vi "Init.vi"(8 "error in (no error)":errorcluster, 10 "Variant":variant, 11 "SpinCoater in":refnum<class "SpinCoater.lvclass">) -> (0 "error out":errorcluster, 3 "SpinCoater out":refnum<class "SpinCoater.lvclass">)   [LabVIEW 2020, in "SpinCoater.lvclass"]
uses:
  <instrlib>/Classes/SpinCoater/SpinCoater.lvclass
  <vilib>/Instr/_visa.llb/VISA Configure Serial Port (Instr).vi
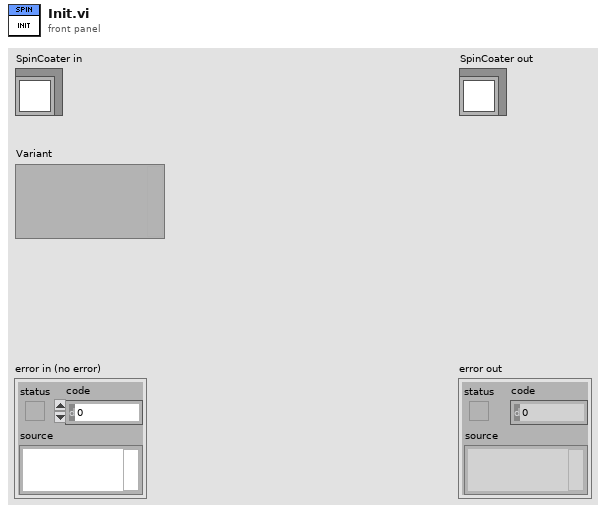
[diagram p1: front panel]
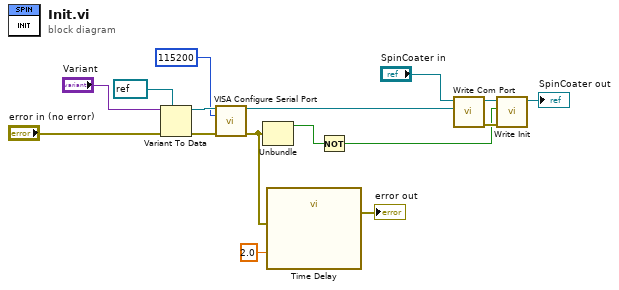
[diagram p0: block diagram]
diagram:
  n1 = Variant To Data(error in="error in (no error)", type=refnum<visa-resource-name> refnum ("VISA resource name"), Variant="Variant") -> (data=w13:refnum<visa-resource-name>, error out=w12:errorcluster)
  n2 = call-poly "VISA Configure Serial Port"("VISA resource name"=w13, "baud rate (9600)"=u32 115200, "error in (no error)"=w12) -> ("VISA resource name out"=w4:refnum<visa-resource-name>, "error out"=w2:errorcluster)  [unwired: 11 in]
  n3 = Unbundle(w2) -> ("status"=w10:bool)  [unwired: 2 out]
  n4 = call "Time Delay"("error in (no error)"=w2, "Delay Time (s)"=2.0) -> ("error out"=→"error out":errorcluster)  [unwired: 9 in]
  n5 = Not(x=w10) -> (.not. x?=w6:bool)
  n6 = call-dynamic "Write Com Port.vi"("Com Port"=w4, "SpinCoater in"="SpinCoater in") -> ("error out"=w7:errorcluster, "SpinCoater out"=w8:refnum<class "SpinCoater.lvclass">)  [unwired: 8 in]
  n7 = call-dynamic "Write Init.vi"("error in (no error)"=w7, "Init"=w6, "SpinCoater in"=w8) -> ("SpinCoater out"=→"SpinCoater out":refnum<class "SpinCoater.lvclass">)  [unwired: 7 in, 1 out]
